vi "Example.vi"() -> ()   [LabVIEW 2019, in "Sig_DI_Simple.lvclass"]
uses:
  Sig_DI_Simple.lvclass
  Database_Postgress_class/Connection Info.ctl
  ConfigJSON_class/ConfigJSON.lvclass
  D:/GIT H4000/H4000/src/ConfigInterface_class/ConfigInterface.lvclass
  MessageAMC_class/MessageAMC.lvclass
  D:/GIT H4000/H4000/src/MessageInterface_class/MessageInterface.lvclass
  Database_Postgress_class/Database_Postgress.lvclass
  D:/GIT H4000/H4000/src/DatabaseInterface_class/DatabaseInterface.lvclass
  Logger_class/Logger.lvclass
  D:/GIT H4000/H4000/src/Proccess_class/Proccess.lvclass
  Sig_DI_Simple.lvclass/Sig_DI_Simple.ctl
  Proccess_class/Proccess.lvclass/Proccess.ctl
  private/write_di_to_db.vi
  Proccess_class/Read TagName.vi
  Proccess_class/Read Logger.vi
  Logger_class/WriteEvent.vi
  <vilib>/NI/AMC/AMC.lvlib
  Proccess_class/Proccess.lvclass
  DatabaseInterface_class/DatabaseInterface.lvclass
panel:
  out "dt":u32
  out "DI":bool
  in  "RAW":bool
  in  "Set RAW 2":bool
  in  "Connection Info":T1={"IP_Address"="localhost", "Port"=5432, "Timeout"=10000, "User"="postgres", "Password"="select12", "Database"="sandbox_controller"}
  in  "stop":bool
  out "error out":errorcluster
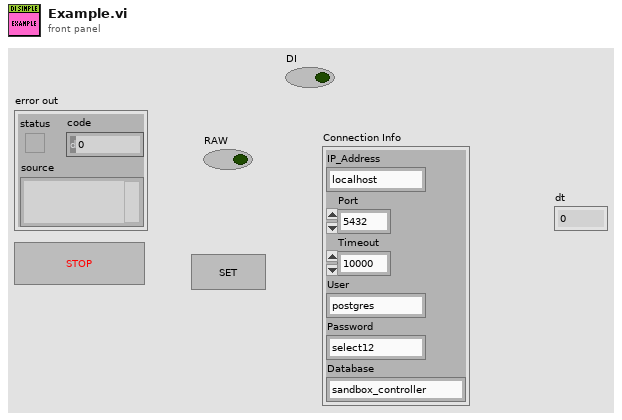
[diagram p1: front panel]
types:
  T1 = typedef "DatabaseInterface.lvclass/Connection Info.ctl" = cluster{"IP_Address":string, "Port":u16, "Timeout":i32, "User":string, "Password":string, "Database":string}
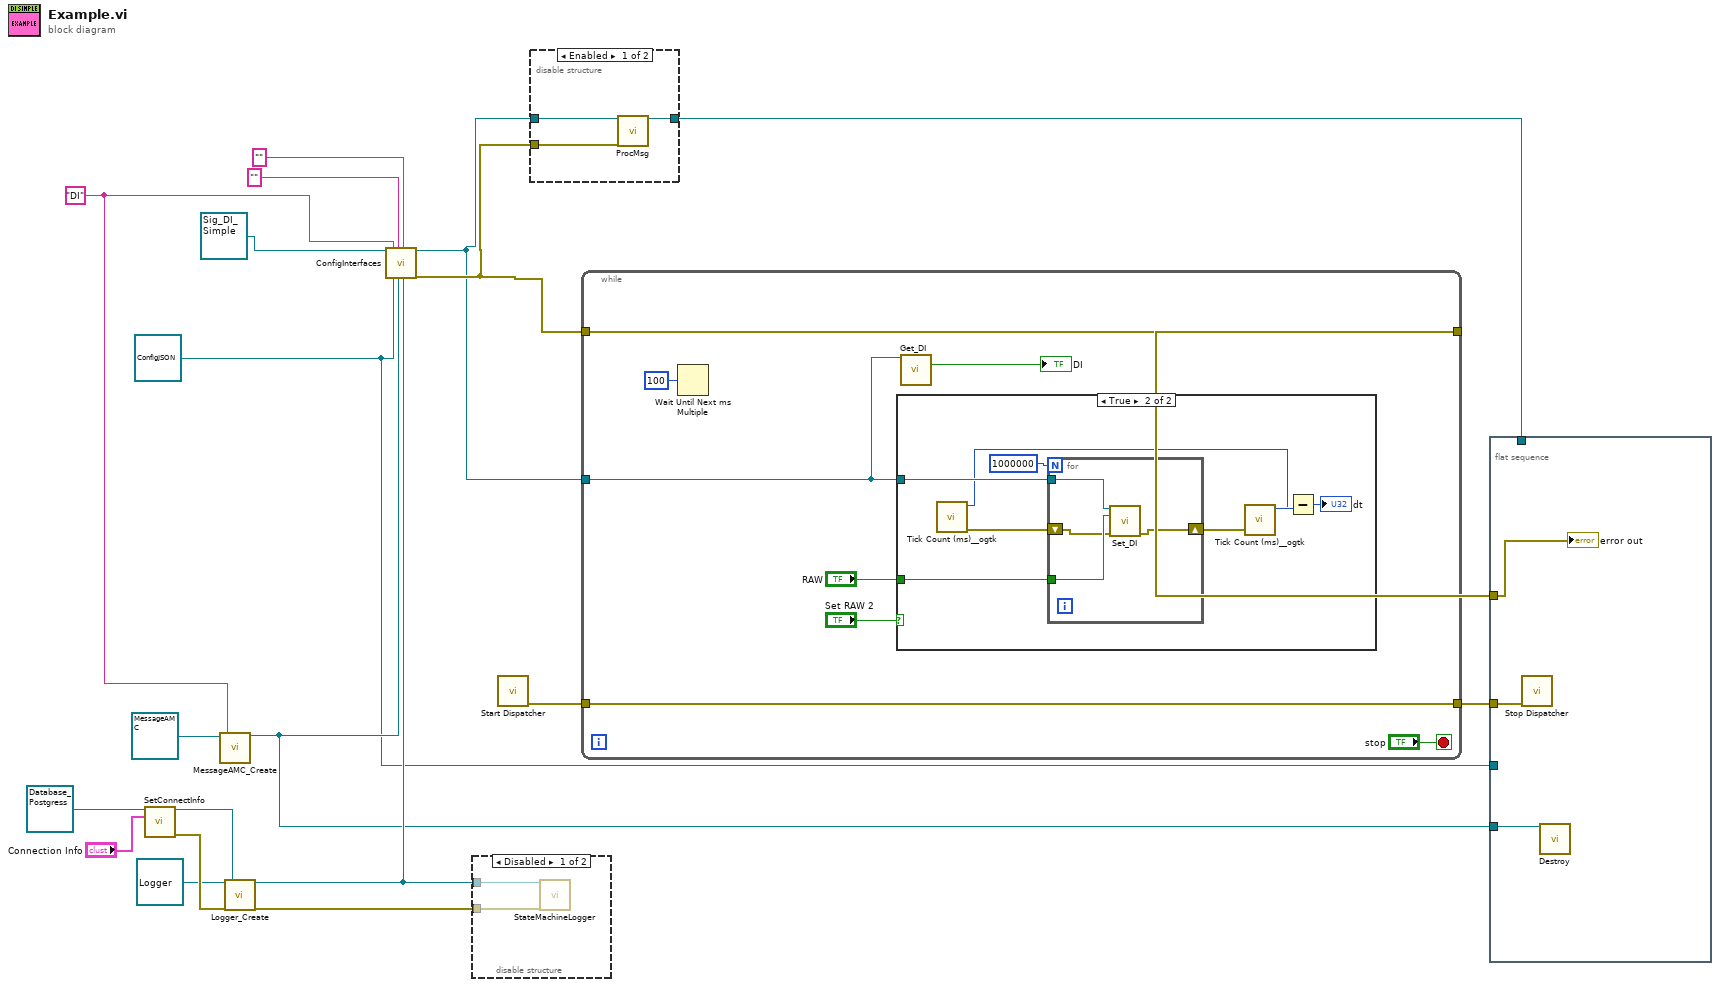
[diagram p0: block diagram]
diagram:
  w2 = refnum<class "ConfigJSON.lvclass"> refnum ("ConfigJSON")
  w5 = "DI" ("Name")
  n1 = call-dynamic "SetConnectInfo.vi"("reference in"=refnum<class "Database_Postgress.lvclass"> refnum, "Connection Info"="Connection Info") -> ("reference out"=w15:refnum<class "Database_Postgress.lvclass">, "error out"=w16:errorcluster)  [unwired: 12 in]
  n2 = call "MessageAMC_Create.vi"("reference in"=refnum<class "MessageAMC.lvclass"> refnum ("MessageAMC"), "message queue name"=w5) -> ("amc"=w3:refnum<class "MessageAMC.lvclass">)  [unwired: 16 in, 1 out]
  n3 = call "Logger_Create.vi"("reference in"=refnum<class "Logger.lvclass"> refnum, "error in (no error)"=w16, "DatabaseInterface"=w15) -> ("reference out"=w4:refnum<class "Logger.lvclass">, "error out"=w12:errorcluster)  [unwired: 15 in]
  n4 = call "ConfigInterfaces.vi"("reference in"=refnum<class "Sig_DI_Simple.lvclass"> refnum ("Sig_DI"), "Name"=w5, "ConfigInterface"=w2, "ParentName"="" ("desc"), "MessageInterface"=w3, "Description"="" ("ParentName"), "Logger"=w4) -> ("reference out"=w9:refnum<class "Sig_DI_Simple.lvclass">, "error out"=w10:errorcluster)  [unwired: 11 in]
  n5 = disable-structure shown="Disabled" {
    disable-tunnel: w12 -> [w22 _]
    disable-tunnel: w4 -> [w21 _]
    frame Disabled {
      n6 = call-dynamic "StateMachineLogger.vi"("reference in"=w21, "error in (no error)"=w22) -> ()  [unwired: 18 in]
    }
    frame Enabled {
    }
  }
  n7 = call <vilib>:"Start Dispatcher.vi"() -> ("error out"=w17:errorcluster)  [unwired: 13 in, 2 out]
  n8 = disable-structure shown="Enabled" {
    disable-tunnel: [w25 w26] -> w11
    disable-tunnel: w10 -> [w24 _]
    disable-tunnel: w9 -> [w23 w26]
    frame Enabled {
      n9 = call "ProcMsg.vi"("reference in"=w23, "error in (no error)"=w24) -> ("reference out"=w25:refnum<class "Sig_DI_Simple.lvclass">)  [unwired: 16 in, 1 out]
    }
    frame Disabled {
    }
  }
  n10 = while {
    tunnel: w10 -> [w34]
    tunnel: [w34] -> w19
    tunnel: [w31] -> w18
    tunnel: w17 -> [w31]
    tunnel: w9 -> [w28]
    stop <- "stop" stop-if-true
    n11 = Wait Until Next ms Multiple(millisecond multiple=u32 100) -> ()  [unwired: 1 out]
    n12 = case shown="True" "Set RAW 2" {
      tunnel: "RAW" -> [_ w42]
      tunnel: w28 -> [_ w41]
      frame False {
      }
      frame True {
        n13 = call <userlib>:"Tick Count (ms)__ogtk.vi"() -> ("error out"=w39:errorcluster, "millisecond timer value"=w36:u32)  [unwired: 10 in]
        n14 = for {
          N: 1000000 -> [_]
          tunnel: w42 -> [w46]
          tunnel: w41 -> [w45]
          shift-right: [w43] -> w38
          shift-left: w39 -> [w44]
          n15 = call "Set_DI.vi"("reference in"=w45, "DI"=w46, "error in (no error)"=w44) -> ("error out"=w43:errorcluster)  [unwired: 11 in, 1 out]
        }
        n16 = call <userlib>:"Tick Count (ms)__ogtk.vi"("error in (no error)"=w38) -> ("millisecond timer value"=w37:u32)  [unwired: 9 in, 1 out]
        n17 = Subtract(x=w37, y=w36) -> (x-y=→"dt":u32)
      }
    }
    n18 = call "Get_DI.vi"("reference in"=w28) -> ("DI"=→"DI":bool)  [unwired: 14 in]
  }
  n19 = flat-sequence {
    tunnel: w19 -> [w49]
    tunnel: w18 -> [w48]
    tunnel: w2 -> [_]
    tunnel: w3 -> [w47]
    tunnel: w11 -> [_]
    frame #0 {
      n20 = call <vilib>:"Stop Dispatcher.vi"("error in"=w48) -> ()  [unwired: 14 in, 1 out]
      n21 = call-dynamic "Destroy.vi"("reference in"=w47) -> ()  [unwired: 17 in, 2 out]
      "error out" <- w49
    }
  }
